vi "Config Scan Variables STMode.vi"(8 "error in":errorcluster, 10 "Mode (Each)":i32(ring) items=["Each", "Inner", "Second", "Third"], 11 "VISA resource name":refnum<visa-resource-name>) -> (0 "error out":errorcluster, 3 "VISA resource name out":refnum<visa-resource-name>)   [LabVIEW 2019, in "Andeen-Hagerling 2700(400 firmware).lvlib"]
doc: "Specifies how the STotal parameter is interpreted."
uses:
  Andeen-Hagerling 2700(400 firmware).lvlib
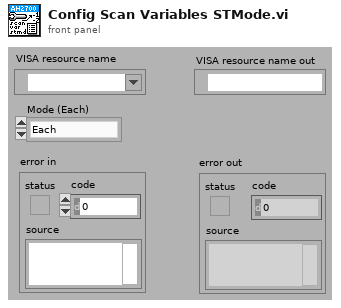
[diagram p1: front panel]
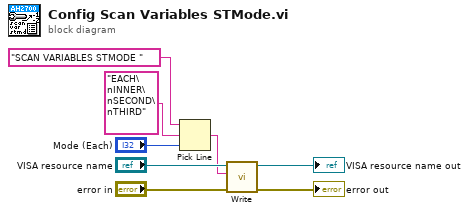
[diagram p0: block diagram]
diagram:
  n1 = Pick Line(string ("")="SCAN VARIABLES STMODE ", multi-line string="EACH\nINNER\nSECOND\nTHIRD", line index="Mode (Each)") -> (output string=w3:string)
  n2 = call "Write.vi"("error in"="error in", "command"=w3, "VISA resource name"="VISA resource name") -> ("error out"=→"error out":errorcluster, "VISA resource name out"=→"VISA resource name out":refnum<visa-resource-name>)  [unwired: 7 in]
